vi "数据显示.vi"() -> ()   [LabVIEW 2018]
panel:
  out "X体横向位移2":dbl
  out "X体横向位移1":dbl
  out "周向转动摩擦力2":dbl
  out "周向转动摩擦力1":dbl
  out "横向拉压力2":dbl
  out "横向拉压力1":dbl
  out "容器压力2":dbl
  out "容器压力1":dbl
  out "管道压力2":dbl
  out "管道压力1":dbl
  in  "选项卡控件 2":enum32{"X体横向位移1", "X体横向位移2"}(tab)
  out "X体横向位移1":dbl(graph)
  out "X体横向位移2":dbl(graph)
  in  "选项卡控件 3":T1(tab)
  out "横向拉压力1":dbl(graph)
  out "横向拉压力2":dbl(graph)
  out "周向转动摩擦力1":dbl(graph)
  out "周向转动摩擦力2":dbl(graph)
  in  "选项卡控件":enum32{"管道压力1", "管道压力2", "容器压力1", "容器压力2"}(tab)
  out "管道气压1":dbl(graph)
  out "管道压力2":dbl(graph)
  out "容器压力1":dbl(graph)
  out "容器压力2":dbl(graph)
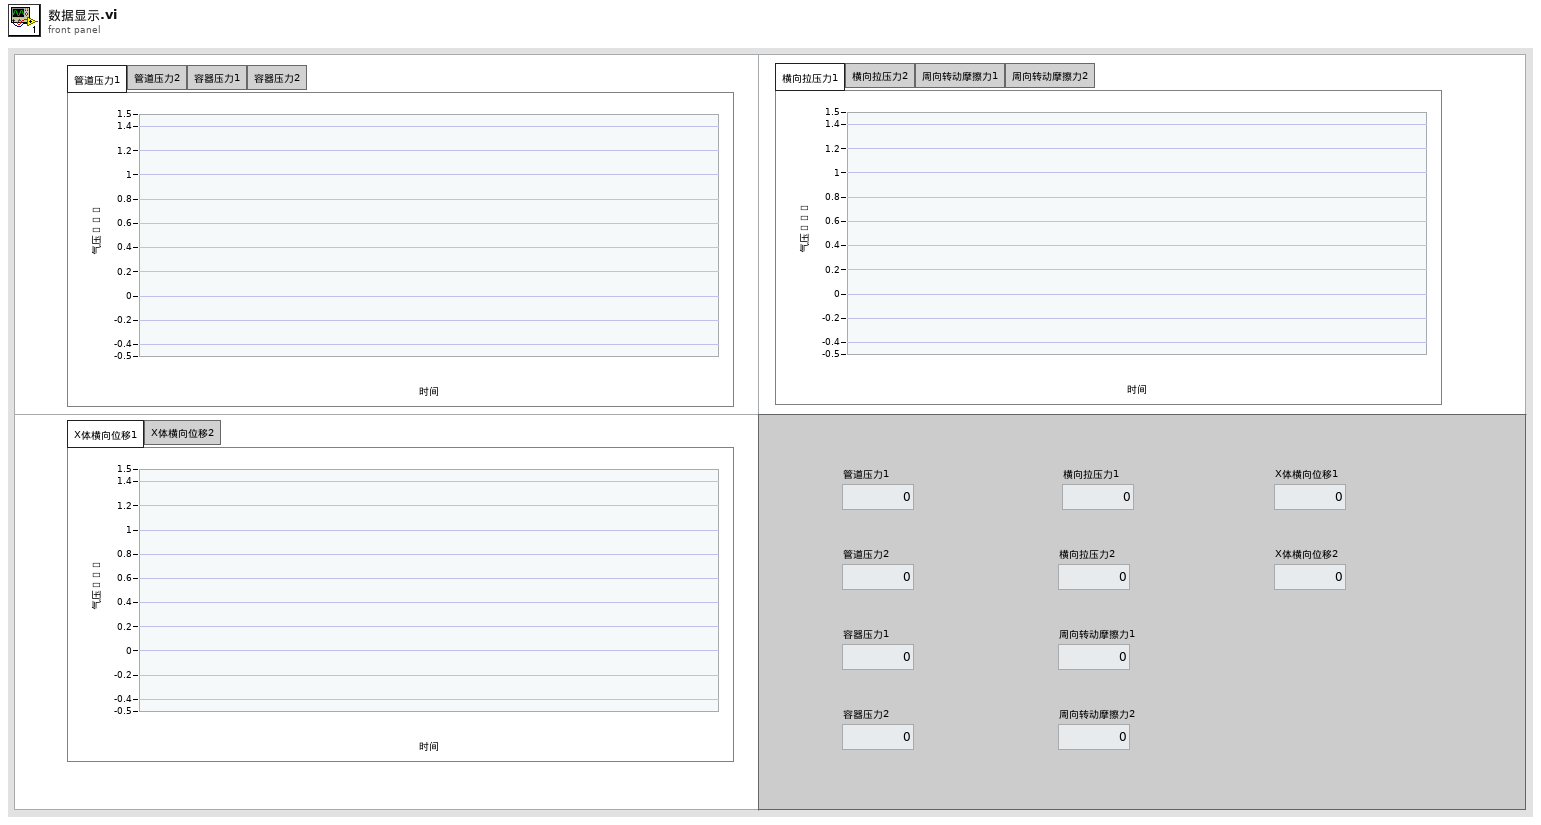
[diagram p1: front panel]
types:
  T1 = enum32{"横向拉压力1", "横向拉压力2", "周向转动摩擦力1", "周向转动摩擦力2"}
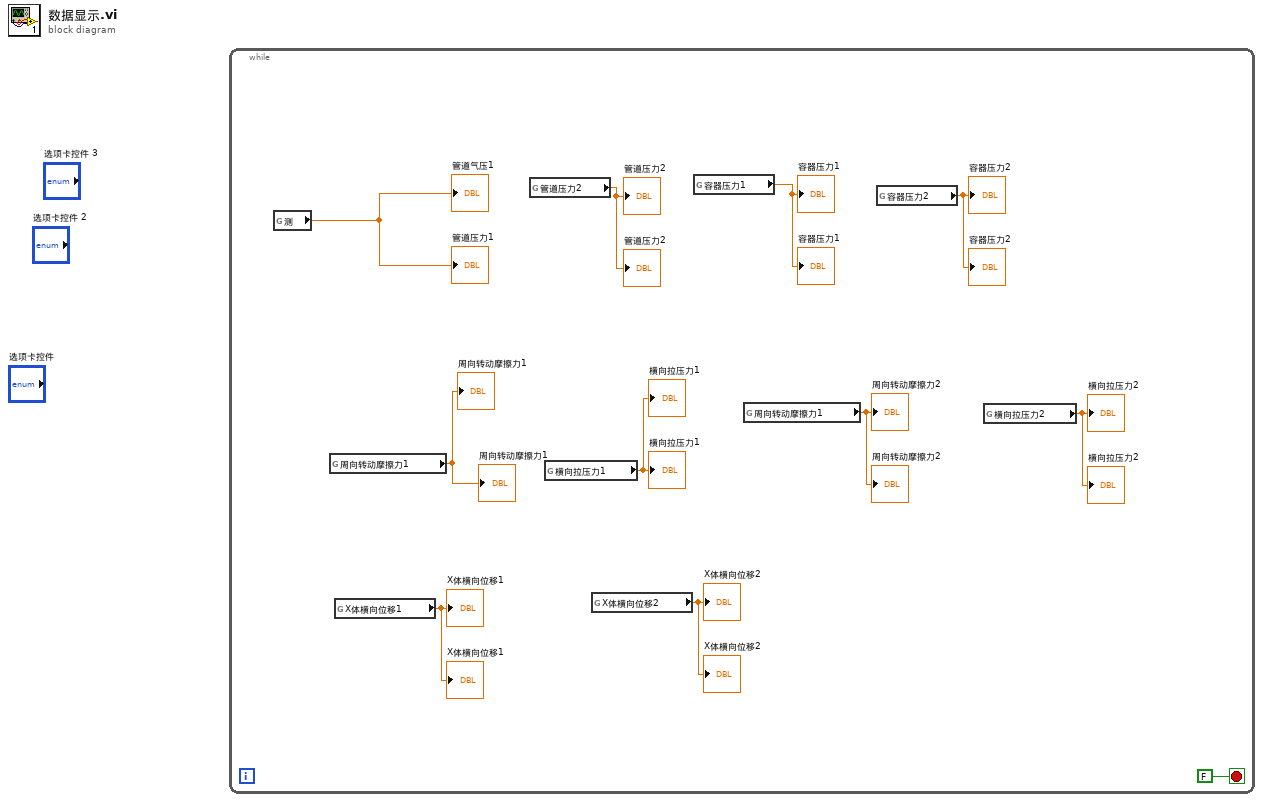
[diagram p0: block diagram]
diagram:
  n1 = while {
    stop <- FALSE stop-if-true
    n2 = global read "全局.vi" "测"() -> (→"管道气压1" →"管道压力1":dbl)
    n3 = global read "全局.vi" "周向转动摩擦力1"() -> (→"周向转动摩擦力1" →"周向转动摩擦力1":dbl)
    n4 = global read "全局.vi" "X体横向位移1"() -> (→"X体横向位移1" →"X体横向位移1":dbl)
    n5 = global read "全局.vi" "管道压力2"() -> (→"管道压力2" →"管道压力2":dbl)
    n6 = global read "全局.vi" "横向拉压力1"() -> (→"横向拉压力1" →"横向拉压力1":dbl)
    n7 = global read "全局.vi" "X体横向位移2"() -> (→"X体横向位移2" →"X体横向位移2":dbl)
    n8 = global read "全局.vi" "容器压力1"() -> (→"容器压力1" →"容器压力1":dbl)
    n9 = global read "全局.vi" "周向转动摩擦力1"() -> (→"周向转动摩擦力2" →"周向转动摩擦力2":dbl)
    n10 = global read "全局.vi" "容器压力2"() -> (→"容器压力2" →"容器压力2":dbl)
    n11 = global read "全局.vi" "横向拉压力2"() -> (→"横向拉压力2" →"横向拉压力2":dbl)
  }
